vi "Set Team Start.vi"(8 "error in (no error)":errorcluster, 9 "Set Team Start":T1, 10 "Team":T2 format="%.0x", 11 "Game in":refnum<class "Game.lvclass">) -> (0 "error out":errorcluster, 3 "Game out":refnum<class "Game.lvclass">)   [LabVIEW 2020, in "SquareBattle.lvlib" / "Game.lvclass"]
uses:
  Game.lvclass
  Team ID.ctl
  Position.ctl
  Game.lvclass/Game.ctl
  SquareBattle.lvlib
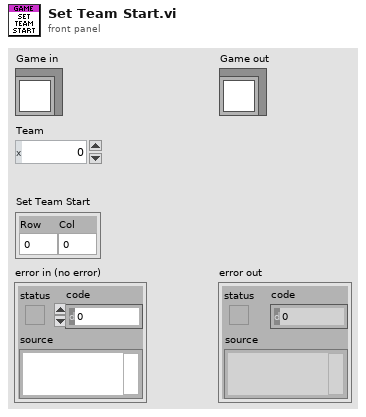
[diagram p1: front panel]
types:
  T1 = typedef "SquareBattle.lvlib/Position.ctl" = cluster{"Row":i32, "Col":i32}
  T2 = typedef "SquareBattle.lvlib/Team ID.ctl" = u32
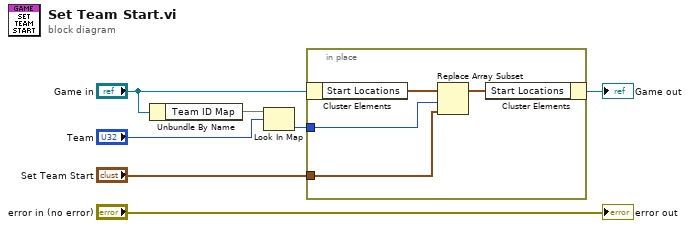
[diagram p0: block diagram]
diagram:
  n1 = Unbundle By Name("Game in") -> ("Team ID Map"=w6:map{T2, i32})
  n2 = Look In Map(map=w6, key="Team") -> (value=w5:i32)  [unwired: 1 in, 1 out]
  n3 = in-place {
    in-place-border: w5 -> [w8]
    in-place-border: "Set Team Start" -> [w9]
    n4 = in-place-cluster #1("Game in") -> ("Start Locations"=w11:T1[])
    n5 = Replace Array Subset(array=w11, new element=w9, index=w8) -> (w10:T1[])
    n6 = in-place-cluster #1("Start Locations"=w10) -> (→"Game out":refnum<class "Game.lvclass">)
  }
  "error out" <- "error in (no error)"
